vi "testSourceTree.vi"() -> ()   [LabVIEW 2015]
panel:
  out "数値: 0から1":dbl
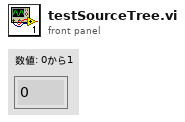
[diagram p1: front panel]
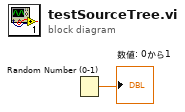
[diagram p0: block diagram]
diagram:
  n1 = Random Number (0-1)() -> (number: 0 to 1=→"数値: 0から1":dbl)
